vi "enqueue.vi"(8 "error in (no error)":errorcluster, 9 "Payload":variant, 10 "states":T1, 11 "queue out":refnum<queue>) -> (0 "error out":errorcluster)   [LabVIEW 2020]
uses:
  message.ctl
  states.ctl
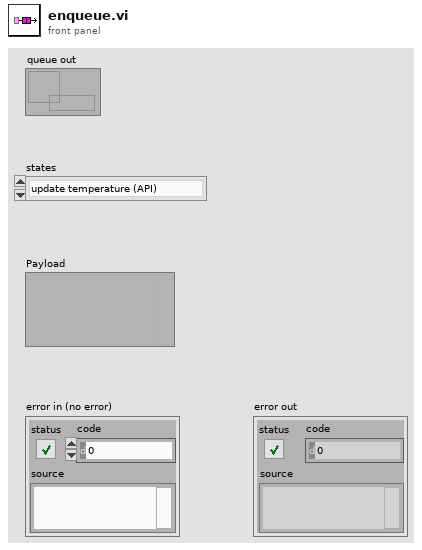
[diagram p1: front panel]
types:
  T1 = typedef "states.ctl" = enum16{"update temperature (API)", "update temperature (User)", "stop"}
  T2 = typedef "message.ctl" = cluster{"states":T1, "Payload":variant}
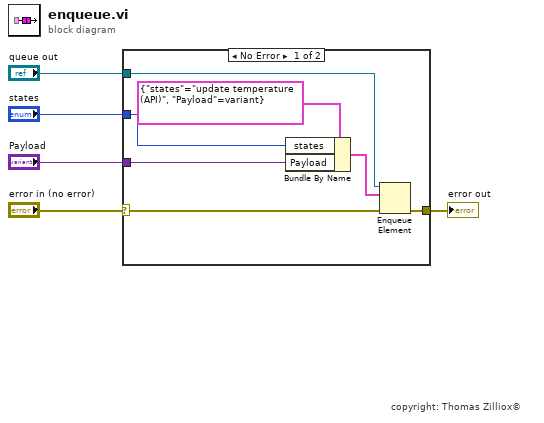
[diagram p0: block diagram]
diagram:
  # "copyright: Thomas Zilliox©"
  n1 = case shown="No Error" "error in (no error)" {
    selector: "error in (no error)" -> [w12 w13]
    tunnel: [w11 w13] -> w4
    tunnel: "queue out" -> [w10 _]
    tunnel: "Payload" -> [w7 _]
    tunnel: "states" -> [w6 _]
    frame No Error {
      n2 = Bundle By Name(cluster=T2 {"states"=enum."update temperature (API)", "Payload"=variant} ("element"), "states"=w6, "Payload"=w7) -> (w8:T2)
      n3 = Enqueue Element(queue=w10, element=w8, error in (no error)=w12) -> (error out=w11:errorcluster)  [unwired: 1 in, 2 out]
    }
    frame Error {
    }
  }
  "error out" <- w4
